vi "Receive Results Object.vi"(8 "error in (no error)":errorcluster, 10 "Results.lvclass":refnum<class "Results.lvclass">, 11 "TestStand Controller in":refnum<class "Controller API.lvclass">) -> (0 "error out":errorcluster, 3 "TestStand Controller out":refnum<class "Controller API.lvclass">)   [LabVIEW 2016, in "Controller API.lvlib" / "Controller API.lvclass"]
uses:
  Controller API.lvclass
  MAL-Framework/user.lib/Common Components/Results/Results.lvclass
  Controller API.lvclass/Controller API.ctl
  MAL-Framework/user.lib/Common Components/Results/Results.lvclass/Results.ctl
  MAL-Framework/user.lib/Common Components/Controller/Controller.lvclass
panel:
  out "Measurement Instance GUID":string
  out "error out 2":errorcluster
  out "found":bool
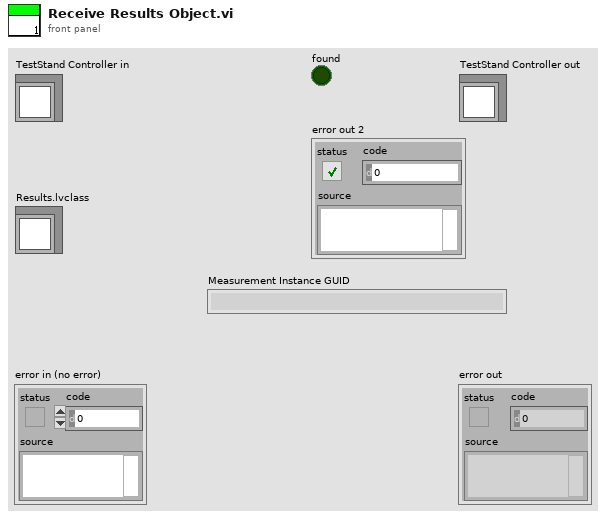
[diagram p1: front panel]
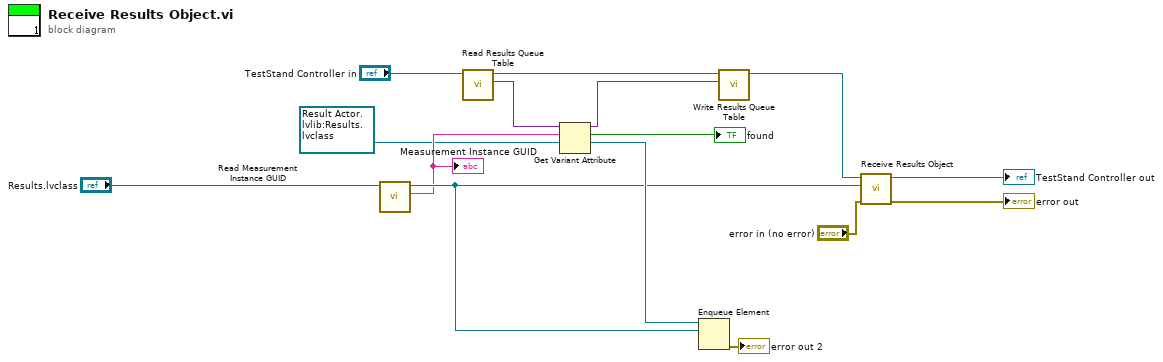
[diagram p0: block diagram]
diagram:
  n1 = call "Read Measurement Instance GUID.vi"("Results in"="Results.lvclass") -> ("Measurement Instance GUID"=w4:string, "Results out"=w5:refnum<class "Results.lvclass">)  [unwired: 8 in, 1 out]
  "Measurement Instance GUID" <- w4
  n2 = call "Read Results Queue Table.vi"("TestStand Controller in"="TestStand Controller in") -> ("Results Queue Table"=w9:variant, "TestStand Controller out"=w11:refnum<class "Controller API.lvclass">)  [unwired: 8 in, 1 out]
  n3 = Get Variant Attribute(Variant=w9, name=w4, default value (empty Variant)=refnum<queue> refnum ("Results Queue")) -> (duplicate Variant=w8:variant, found=→"found":bool, value=w7:refnum<queue>)  [unwired: 1 in, 1 out]
  n4 = Enqueue Element(queue=w7, element=w5) -> (error out=→"error out 2":errorcluster)  [unwired: 2 in, 2 out]
  n5 = call "Write Results Queue Table.vi"("Results Queue Table"=w8, "TestStand Controller in"=w11) -> ("TestStand Controller out"=w10:refnum<class "Controller API.lvclass">)  [unwired: 8 in, 1 out]
  n6 = call-parent "Receive Results Object.vi"("error in (no error)"="error in (no error)", "Results.lvclass"=w5, "Controller in"=w10) -> ("error out"=→"error out":errorcluster, "Controller out"=→"TestStand Controller out":refnum<class "Controller API.lvclass">)  [unwired: 7 in]
